vi "zmq_socket.vi"(4 "error in":errorcluster, 5 "linger (ms)":i32, 6 "socket type":T1, 7 "context in":refnum<class "zmq_context.lvclass">) -> (0 "error out":errorcluster, 2 "socket out":refnum<class "zmq_socket.lvclass">, 3 "context out":refnum<class "zmq_context.lvclass">)   [LabVIEW 2019, in "zeromq.lvlib" / "zmq_context.lvclass"]
doc: "Create a socket of flavour <b>socket type</b> in context <b>ctx in</b> and linger time <b>linger</b> milliseconds (time permitted after zmq_term to finish queued operations).\n\nNote that ZeroMQ creates sockets with infinite linger (ZMQ_LINGER) by default, which is undesirable in a managed environment like LabVIEW since it hangs the parent process. But set it to -1 should infinite linger be required.\n\nDetailed API documentation: http://api.zeromq.org/3-2:zmq-socket"
uses:
  zmq_context.lvclass
  socket_type.ctl
  zmq_socket.lvclass
  zmq_context.lvclass/zmq_context.ctl
  <vilib>/Utility/error.llb/Error Cluster From Error Code.vi
  zeromq.lvlib
panel:
  # "ØMQ"
  # "labview"
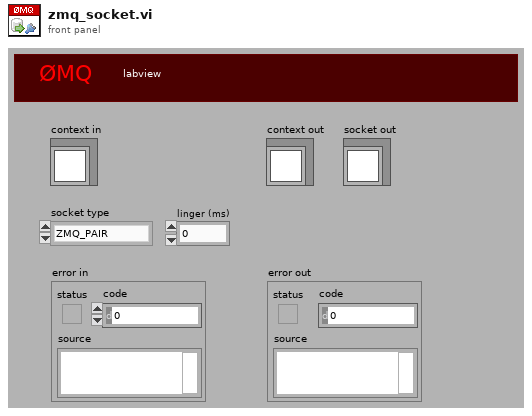
[diagram p1: front panel]
types:
  T1 = typedef "zeromq.lvlib/socket_type.ctl" = enum8{"ZMQ_PAIR", "ZMQ_PUB", "ZMQ_SUB", "ZMQ_REQ", "ZMQ_REP", "ZMQ_DEALER", "ZMQ_ROUTER", "ZMQ_PULL", "ZMQ_PUSH", "ZMQ_XPUB", "ZMQ_XSUB"}
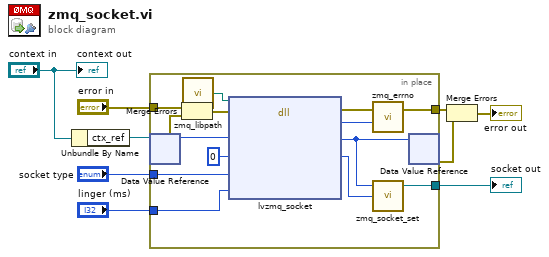
[diagram p0: block diagram]
diagram:
  n1 = Unbundle By Name("context in") -> ("ctx_ref"=w3:refnum<data-value>)
  n2 = in-place {
    in-place-border: "error in" -> [w23]
    in-place-border: "socket type" -> [w22]
    in-place-border: "linger (ms)" -> [w19]
    in-place-border: [w18] -> w5
    in-place-border: [w16] -> w4
    n3 = in-place-dvr #1(w3) -> (w15:u64, w10:errorcluster)
    n4 = Merge Errors(w23, w10) -> (w11:errorcluster)
    n5 = call "zmq_libpath.vi"() -> ("path"=w12:path)
    n6 = dll-call lib="?" fn="lvzmq_socket"(path in=w12, error in=w11, "ctx_obj"=w15, "sock_obj"=u64 0, "type"=w22, "linger"=w19) -> (error out=w21:errorcluster, "return type"=w20:i32, "ctx_obj"=w14:u64, "sock_obj"=w17:u64)  [unwired: 3 in, 1 out]
    n7 = call "zmq_errno.vi"("retval"=w20, "error in"=w21) -> ("error out"=w18:errorcluster)  [unwired: 1 out]
    n8 = call "zmq_socket_set.vi"("socket"=w17, "context"=w14) -> ("socket out"=w16:refnum<class "zmq_socket.lvclass">)  [unwired: 2 in, 1 out]
    n9 = in-place-dvr #1(w14) -> (w1:errorcluster)  [unwired: 1 out]
  }
  "socket out" <- w4
  n10 = Merge Errors(w5, w1) -> (→"error out":errorcluster)
  "context out" <- "context in"
